vi "GetMultipleInstruments.vi"(8 "error in (no error)":errorcluster, 10 "Parameter":string[](array[string]), 11 "ByteGSWebAPI-V0 in":refnum<class "ByteGSWebAPI-V0.lvclass">) -> (0 "error out":errorcluster, 2 "MultipleInstruments":T1, 3 "ByteGSWebAPI-V0 out":refnum<class "ByteGSWebAPI-V0.lvclass">, 4 "MultipleBody":string[](array[string]), 6 "MultipleHeaders":string[](array[string]))   [LabVIEW 2019, in "ByteGSWebAPI.lvlib" / "ByteGSWebAPI-V0.lvclass"]
uses:
  ByteGSWebAPI-V0.lvclass
  Cntrls/MultipleInstruments.ctl
  Cntrls/SingleInstrument.ctl
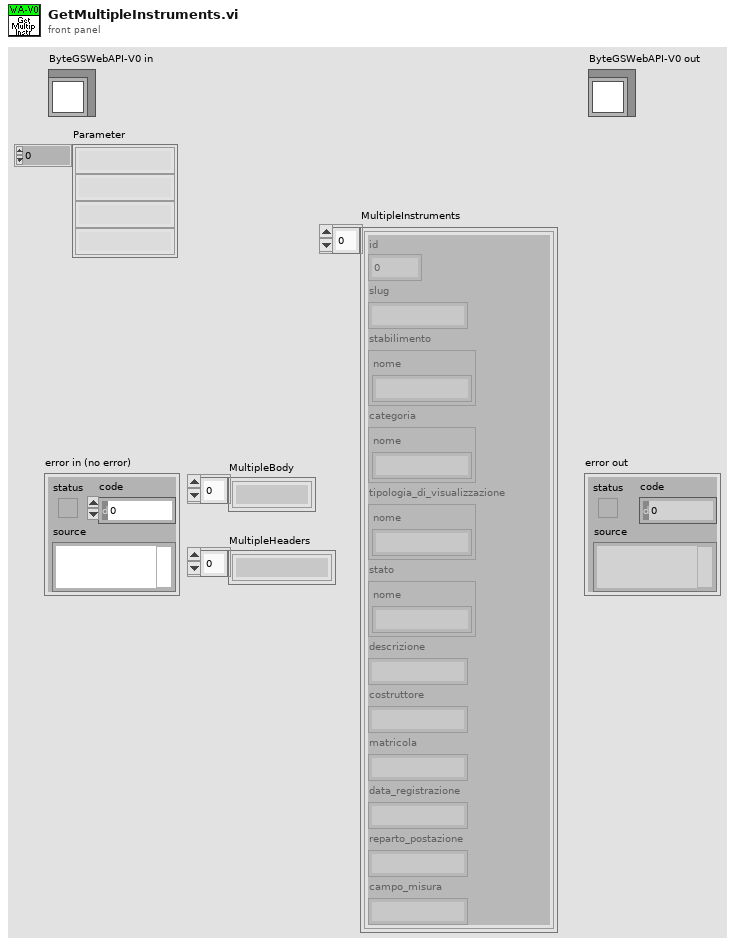
[diagram p1: front panel]
types:
  T1 = typedef "ByteGSWebAPI.lvlib/ByteGSWebAPI-V0.lvclass/MultipleInstruments.ctl" = T2[]
  T2 = typedef "ByteGSWebAPI.lvlib/ByteGSWebAPI-V0.lvclass/SingleInstrument.ctl" = cluster{"id":i32, "slug":string, "stabilimento":cluster{"nome":string}, "categoria":cluster{"nome":string}, "tipologia_di_visualizzazione":cluster{"nome":string}, "stato":cluster{"nome":string}, "descrizione":string, "costruttore":string, "matricola":string, "data_registrazione":string, "reparto_postazione":string, "campo_misura":string}
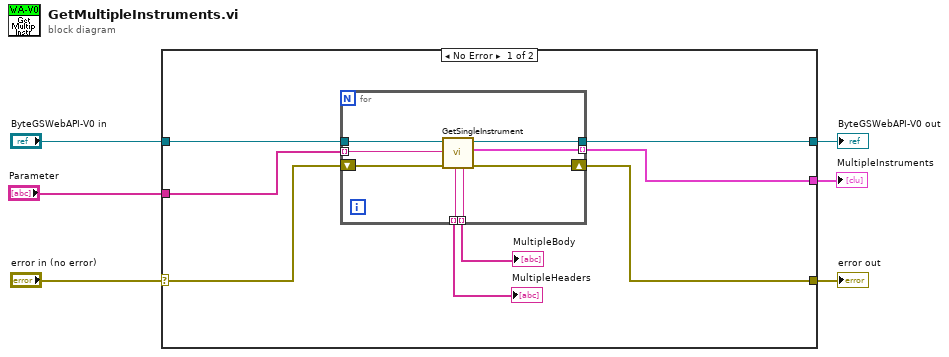
[diagram p0: block diagram]
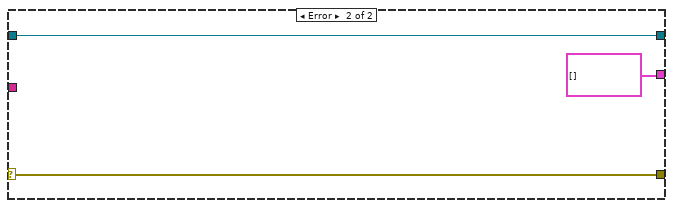
[diagram p2: hidden frame]
diagram:
  n1 = case shown="No Error" "error in (no error)" {
    selector: "error in (no error)" -> [w11 w25]
    tunnel: [w10 w25] -> w5
    tunnel: [w14 w24] -> w3
    tunnel: "ByteGSWebAPI-V0 in" -> [w13 w24]
    tunnel: "Parameter" -> [w12 _]
    tunnel: [w7 T2[] []] -> w1
    frame No Error {
      n2 = for {
        tunnel: w13 -> [w22]
        tunnel: [w21] -> w14
        tunnel: w12 -> [w20] mode=indexing
        shift-right: [w18] -> w10
        shift-left: w11 -> [w19]
        tunnel: [w17] -> w9 mode=indexing
        tunnel: [w16] -> w8 mode=indexing
        tunnel: [w15] -> w7 mode=indexing
        n3 = call-dynamic "GetSingleInstrument.vi"("error in (no error)"=w19, "Parameter"=w20, "ByteGSWebAPI-V0 in"=w22) -> ("error out"=w18:errorcluster, "JSON_Data"=w15:T2, "ByteGSWebAPI-V0 out"=w21:refnum<class "ByteGSWebAPI-V0.lvclass">, "body"=w16:string, "headers"=w17:string)  [unwired: 4 in]
      }
      "MultipleHeaders" <- w9
      "MultipleBody" <- w8
    }
    frame Error {
    }
  }
  "error out" <- w5
  "ByteGSWebAPI-V0 out" <- w3
  "MultipleInstruments" <- w1
